vi "Toggle2.vi"(1 "In 2":bool) -> (0 "Out 2":bool)   [LabVIEW 2020]
uses:
  <vilib>/ptbypt/NI_PtbyPt.lvlib
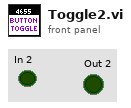
[diagram p1: front panel]
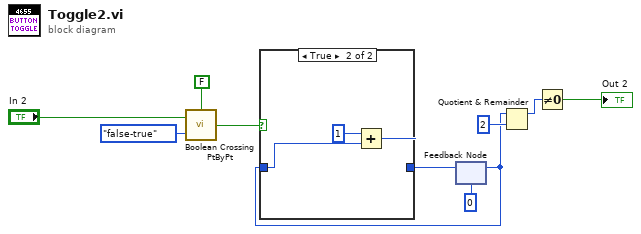
[diagram p0: block diagram]
diagram:
  n1 = call <vilib>:"Boolean Crossing PtByPt.vi"("initialize"=FALSE, "direction"=enum16{"either", "false-true", "true-false"}."false-true", "input"="In 2") -> ("crossing"=w9:bool)
  n2 = feedback #1(0) -> (w3:i32)
  n3 = case shown="True" w9 {
    tunnel: w3 -> [w11 w14]
    tunnel: [w11 w12] -> w4
    frame False {
    }
    frame True {
      n4 = Add(x=1, y=w14) -> (x+y=w12:i32)
    }
  }
  n5 = feedback-in #1(w4) -> ()
  n6 = Quotient & Remainder(x=w3, y=2) -> (x-y*floor(x/y)=w7:i32)  [unwired: 1 out]
  n7 = Not Equal To 0?(x=w7) -> (x != 0?=→"Out 2":bool)
